vi "RPA.vi"(0 "System no.":i32=1 min=1 max=4 step=1, 2 "Affected axes":string[](array[string]), 4 "Parameter no. format \n(Decimal: FALSE)":bool, 5 "error in":errorcluster, 6 "Parameter to restore":i32[](array[numeric]), 7 "Parameter to restore (hex)":u32[](array[numeric]) format="%.0x") -> (14 "Controller error":bool, 19 "error out":errorcluster)   [LabVIEW 2020]
doc: "Replaces the current values of the given parameters to restore for Affected axes in the controller RAM with the values from non-volatile memory, waits 5000 ms and queries ERR?. For axis-related parameters, Affected axes is the axis name, for piezo- or sensor-related parameters, the channel number, otherwise a parameter-related code. If parameter no. is in decimal format, use Parameter to restore input, for hexadecimal parameter numbers use Parameter to restore (hex) input and switch Parameter no. format to TRUE. Do not mix decimal and hex. parameter numbers in one call. See GCS DLL manual for available parameter numbers. If Affected axes is an empty array, RPA is sent without axis (item) and parameter specification and controller restores all values for all axes (items). Controller error is TRUE if selected system reports error code not equal to 0. \n\nE-710, E-761: If Affected axes = empty array, all parameters for all axes are restored. Parameter no. format is TRUE (hex.). Use HPA?.vi to get valid parameter numbers or see the E7XX_GCS_DLL Manual.\n\nC-413, E-517, E-518, E-712, E-725, E-727, E-753, E-754, E-755: If Affected axes = empty array, all parameters for all axes are restored. Parameter no. format is TRUE (hex.). Use HPA?.vi to get valid parameter numbers or see user manual.\n\nC-867, C-877, C-884, E-709, E-861, E-870, E-871, E-873, E-874, Mercury_GCS: You can reset either all parameters or one single parameter with RPA. If Affected axes = empty array, all parameters for all axes are restored. Parameter no. format is TRUE (hex.). Use HPA?.vi to get valid parameter numbers or see user manual."
panel:
  # "Replaces the current values of the given parameters to restore for \"Affected axes\" in the controller RAM with the values from \nnon-volatile memory, waits 5000 ms and queries ERR?. If parameter no. is in decimal format, use \"Parameter to restore\" input, \nfor hexadecimal parameter numbers use \"Parameter to restore (hex)\" input and switch \"Parameter no. format\" to TRUE.  Do not \nmix decimal and hex. parameter numbers in one call. See GCS DLL manual for available parameter numbers. If \"Affected axes\" \nis an empty array, RPA is sent without axis and parameter specification and controller restores all values for all axes."
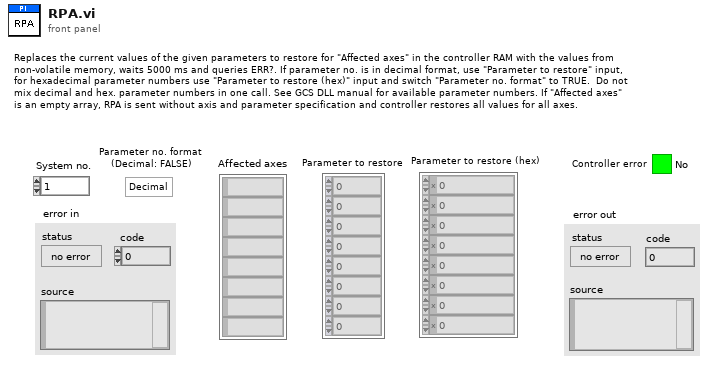
[diagram p1: front panel]
types:
  T1 = enum16{"Disable error check", "Force error check", "Use global settings"}
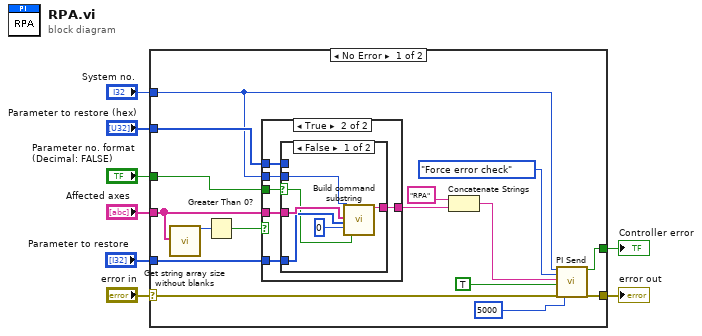
[diagram p0: block diagram]
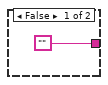
[diagram p2: hidden frame]
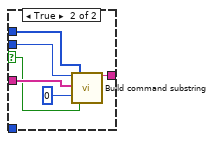
[diagram p3: hidden frame]
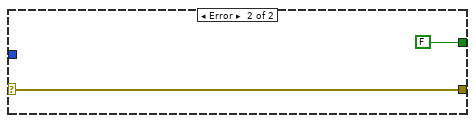
[diagram p4: hidden frame]
diagram:
  n1 = case shown="No Error" "error in" {
    selector: "error in" -> [w14 w44]
    tunnel: [w12 w44] -> w8
    tunnel: "System no." -> [w15 _]
    tunnel: [w11 FALSE ("Controller error")] -> w6
    tunnel: "Affected axes" -> [w21 _]
    tunnel: "Parameter to restore" -> [w22 _]
    tunnel: "Parameter to restore (hex)" -> [w17 _]
    tunnel: "Parameter no. format \n(Decimal: FALSE)" -> [w16 _]
    frame No Error {
      n2 = call "Get string array size without blanks.vi"("String array"=w21) -> ("Corrected array size"=w20:i32)  [unwired: 18 out]
      n3 = Greater Than 0?(x=w20) -> (x > 0?=w19:bool)
      n4 = case shown="True" w19 {
        tunnel: w21 -> [_ w31]
        tunnel: w22 -> [_ w30]
        tunnel: ["" ("Command substring") w29] -> w18
        tunnel: w17 -> [_ w28]
        tunnel: w16 -> [_ w27]
        tunnel: w15 -> [_ w26]
        frame False {
        }
        frame True {
          n5 = case shown="False" w27 {
            selector: w27 -> [w32 w38]
            tunnel: w31 -> [w36 w42]
            tunnel: w30 -> [w35 _]
            tunnel: [w34 w41] -> w29
            tunnel: w28 -> [_ w40]
            tunnel: w26 -> [w33 w39]
            frame False {
              n6 = call "Build command substring.vi"("System no."=w33, "Affected axes"=w36, "Parameters"=w35, "No. of digits"=i16 0, "Parameter no. format \n(Decimal: FALSE)"=w32) -> ("Command substring"=w34:string)  [unwired: 2 in, 12 out]
            }
            frame True {
              n7 = call "Build command substring.vi"("System no."=w39, "Affected axes"=w42, "No. of digits"=i16 0, "Parameters (hex)"=w40, "Parameter no. format \n(Decimal: FALSE)"=w38) -> ("Command substring"=w41:string)  [unwired: 2 in, 12 out]
            }
          }
        }
      }
      n8 = Concatenate Strings("RPA", w18) -> (w23:string)
      n9 = call "PI Send.vi"("System no."=w15, "Error check settings"=T1."Force error check", "String to send"=w23, "Attach termination char.?"=TRUE ("Attach Linefeed?"), "error in"=w14, "Delay before error check (ms)"=u32 5000 ("millisecond timer value")) -> ("Controller error"=w11:bool, "error out"=w12:errorcluster)  [unwired: 12 out]
    }
    frame Error {
    }
  }
  "error out" <- w8
  "Controller error" <- w6
